vi "SubVI ATI.vi"() -> ()   [LabVIEW 2021]
uses:
  ctlSeqFNs_SubVI ATI.ctl
  ctlPkgATI.ctl
  ctlTrialState.ctl
  ctlSeqFNs.ctl
  ctlSeqFNs_SubVI PhaseSpace.ctl
  <vilib>/Analysis/Matrix/Datatypes/RealMatrix.ctl
  ctlRecording.ctl
  <vilib>/DAQmx/read.llb/DAQmx Read (Analog 2D DBL NChan NSamp).vi
  <vilib>/Analysis/baseanly.llb/Real A x B.vi
  <vilib>/Analysis/baseanly.llb/Mean (DBL).vi
  GLOBAL -MAIN.vi
  <vilib>/DAQmx/configure/trigger.llb/DAQmx Start Trigger (Digital Edge).vi
  <vilib>/DAQmx/miscellaneous.llb/DAQmx Fill In Error Info.vi
  <vilib>/Analysis/Matrix/Numeric/Conversions/Array To Matrix - RA2.vi
  <vilib>/Analysis/Matrix/Numeric/Conversions/Matrix To Array - RM.vi
  <vilib>/Analysis/Matrix/NI_Matrix.lvlib
  <resource>/objmgr/daqmx.rc
  <vilib>/Analysis/NI_AALBase.lvlib
panel:
  out "ATI plot 4":dbl[][](graph)
  out "ATI plot 3":dbl[][](graph)
  out "ATI plot 2":dbl[][](graph)
  out "ATI plot 1":dbl[][](graph)
  in  "Calib Files - TShape":path[](array[path])=[path "C:/ATI Calib files/FT8610.cal", path "C:/ATI Calib files/FT9244.cal"]
  in  "UShape?":bool
  out "Hz":dbl(graph)
  in  "Calib files - UShape":T1={"Calibration Files 1"=[path "Z:/Yen/ATI Calib files/FT8610.cal"], "Calibration Files 2"=[path "Z:/Yen/ATI Calib files/FT9244.cal"], "Calibration Files 3"=[path "Z:/Yen/ATI Calib files/FT5076.cal"], "Calibration Files 4"=[path "Z:/Yen/ATI Calib files/FT11787.cal"]}
  out "Bias":dbl[][](array[numeric]) format="%#.2f"
  in  "Bias":bool
  in  "Calib":bool
  out "save file":path
  in  "Read Cycle Time (s)":dbl=0.1 min=0.01 max=10.0 step=0.01 format="%.2f"
  out "recording?":bool
  in  "STOP":bool
  # "Parallel SubVI ATI"
  # "Acquires ATI data and Trigger signal\nSaves TDMS file."
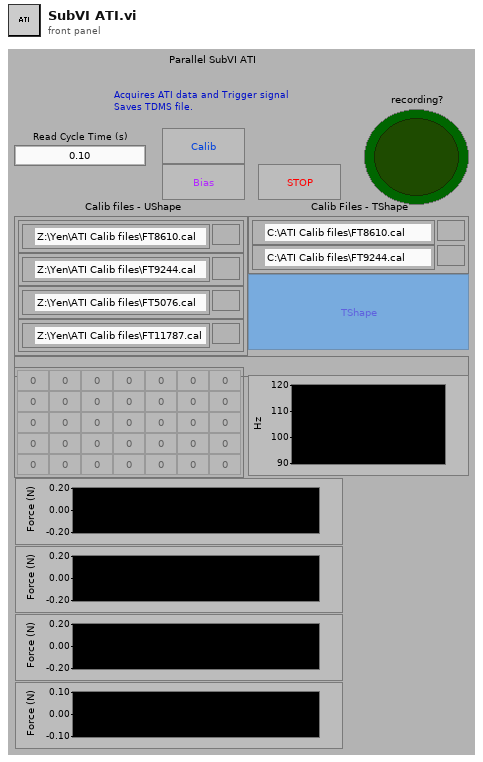
[diagram p1: front panel]
types:
  T1 = cluster{"Calibration Files 1":path[], "Calibration Files 2":path[], "Calibration Files 3":path[], "Calibration Files 4":path[]}
  T2 = typedef "ctlPkgATI.ctl" = cluster{"VIRef":refnum<vi>, "ATI":refnum<k34>, "tick ini":i64, "Trigger events":T3, "connected to server?":bool, "MAIN":refnum<queue>, "PhaseSpace":refnum<queue>, "recording?":bool, "Bias":dbl[][], "DAQmx":refnum<k21>[], "CalibMatrix":cluster{"Real Matrix":T4}[], "Data":cluster{dbl[][]}[], "tick pre":i64, "ATI Ch Names 1":string[], "ATI Ch Names 2":string[], "ATI Ch Names 3":string[], "ATI Ch Names 4":string[], "UShape?":bool}
  T3 = typedef "ctlTrialState.ctl" = enum16{"no events", "ready", "start", "hold", "stop", "end"}
  T4 = typedef "NI_Matrix.lvlib/RealMatrix.ctl" = dbl[][]
  T5 = typedef "ctlSeqFNs_SubVI ATI.ctl" = enum16{"INITIALIZE", "SET HANDLE", "IDLE", "READY", "SEND2MAIN", "CALIB Load", "BIAS", "TRIGGER", "END", "ERROR", "EXIT"}
  T6 = typedef "ctlSeqFNs.ctl" = enum16{"INITIALIZE MAIN", "UpdateProtocol", "UpdateBlockInfo", "UpdatePath", "INITIALIZE Sub", "IDLE", "Bias", "Ready", "RepeatTrial", "Events", "Get PS bias", "Get PhaseSpace", "Get ATI", "Finish", "End PhaseSpace", "End ATI", "ERROR", "EXIT"}
  T7 = typedef "ctlSeqFNs_SubVI PhaseSpace.ctl" = enum16{"INITIALIZE", "IDLE", "BIAS", "READY", "SEND2MAIN", "LOG2TDMS", "TRIGGER", "END", "ERROR", "EXIT"}
  T8 = enum16{"ALIGN -CENTER", "ALIGN -TOP LEFT", "ALIGN -AS IS", "ALIGN -CUSTOM"}
  T9 = typedef "ctlRecording.ctl" = cluster{"recording?":bool, "tdms file":refnum<k34>}
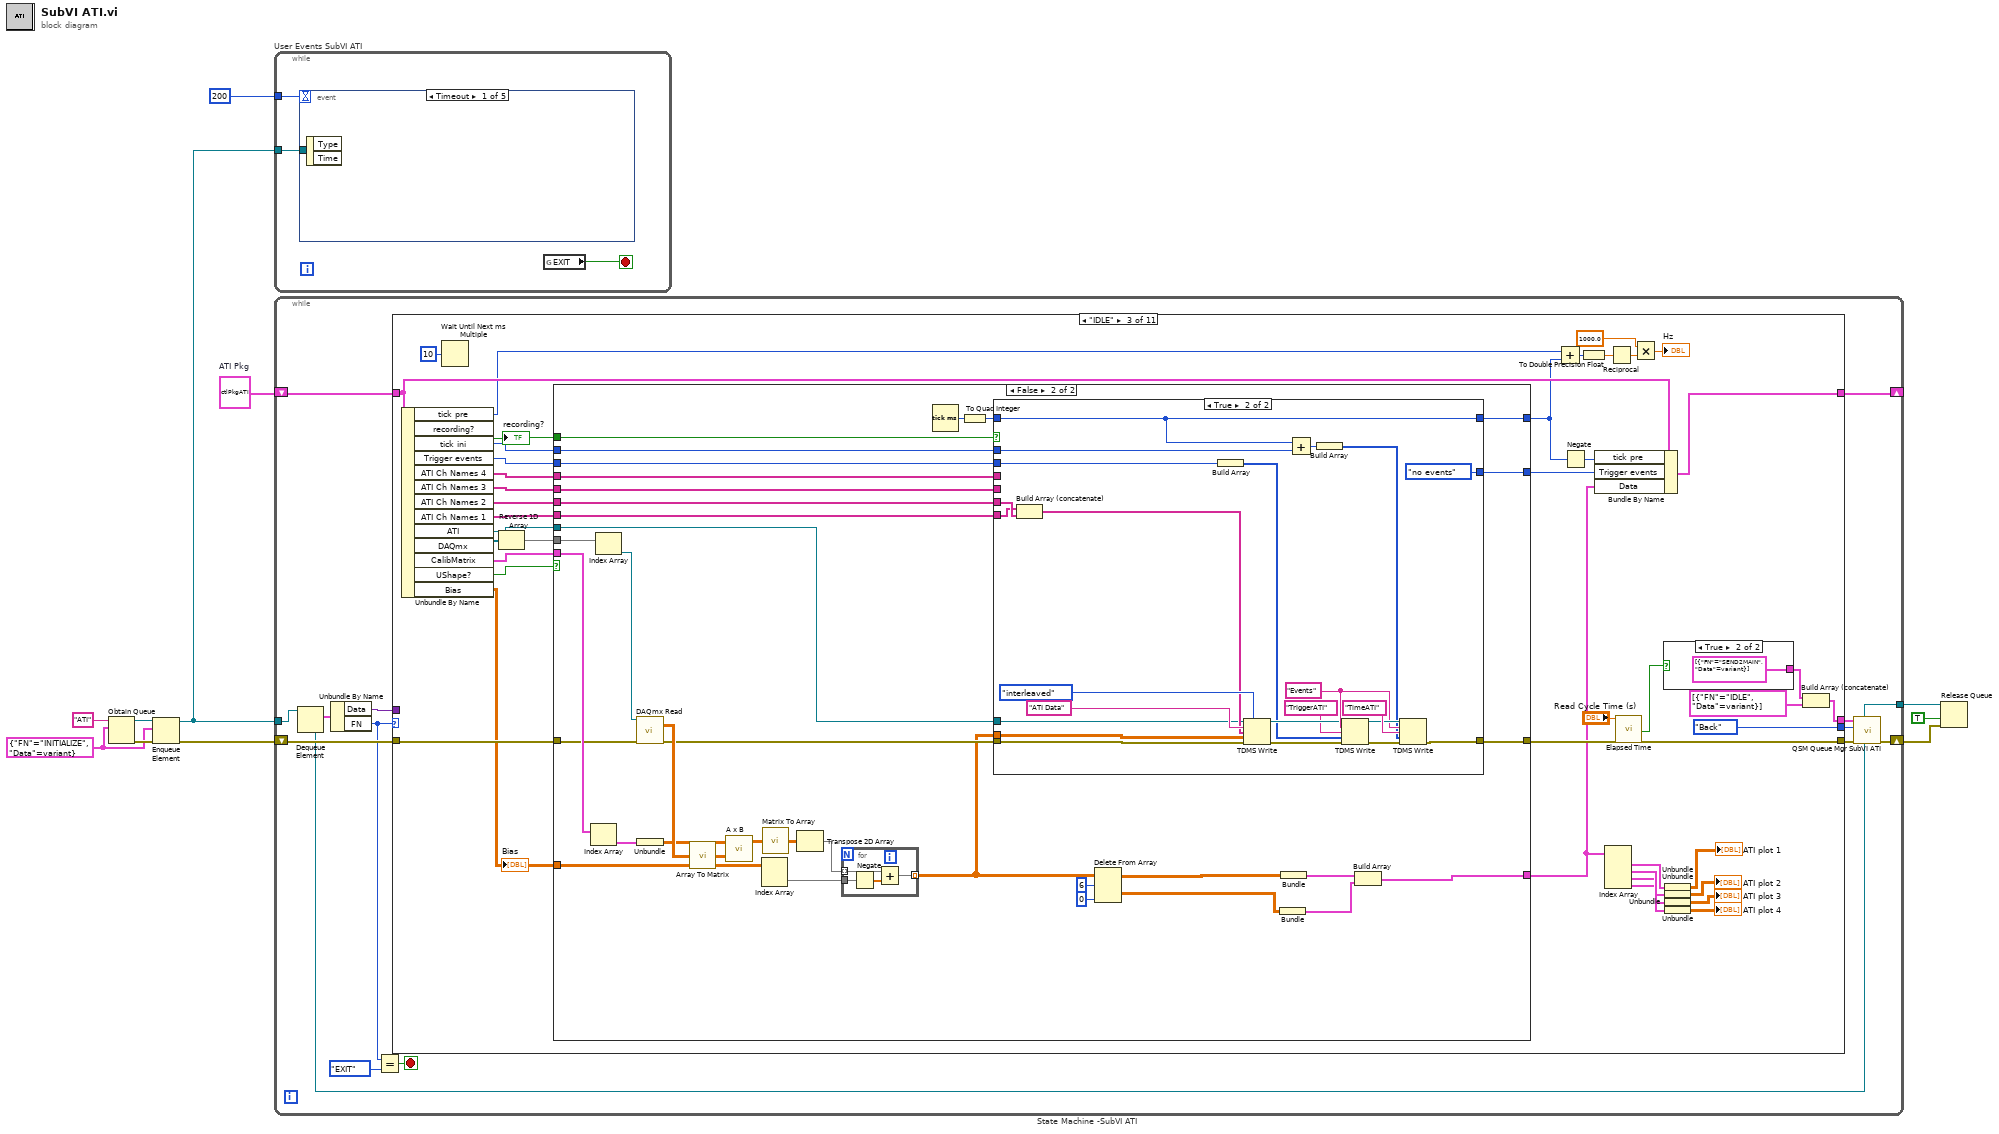
[diagram p0: block diagram]
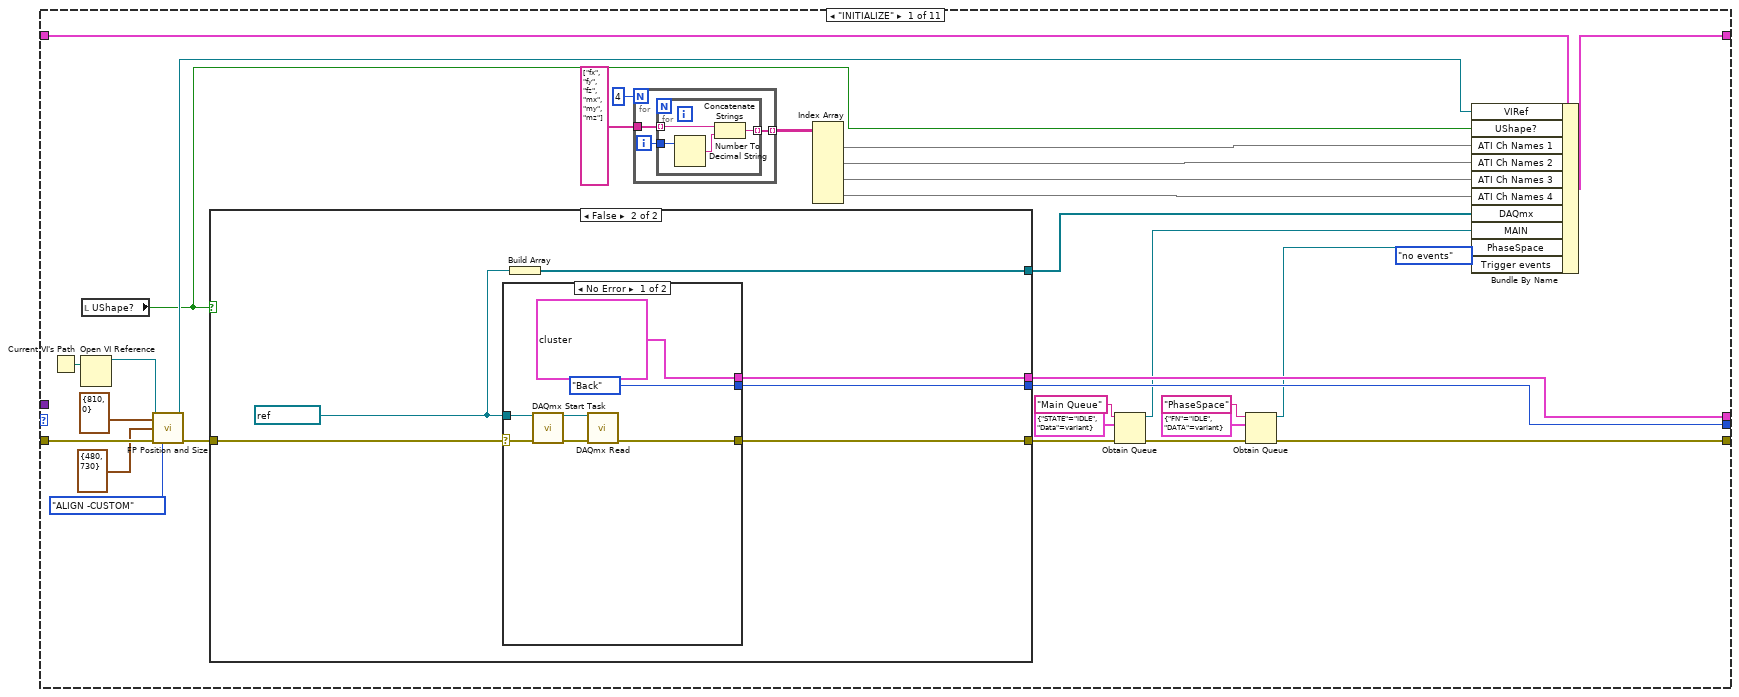
[diagram p2: hidden frame]
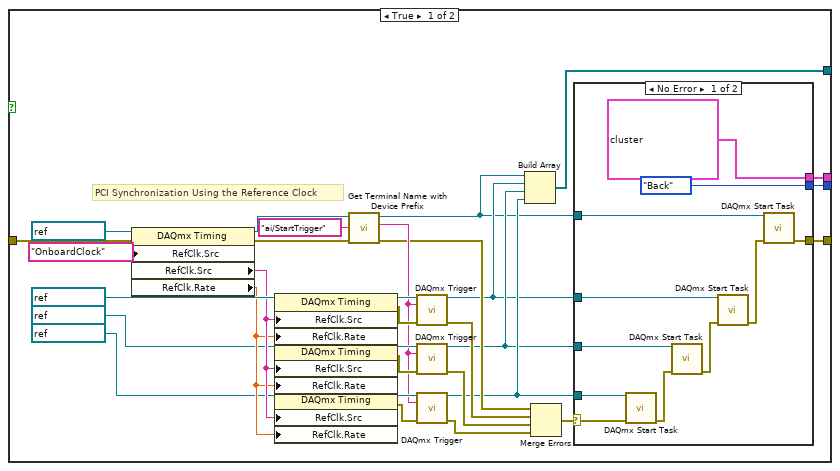
[diagram p3: hidden frame]
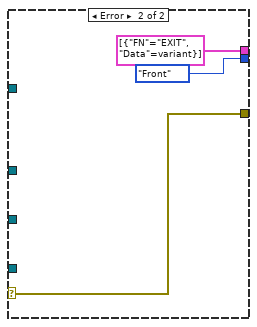
[diagram p4: hidden frame]
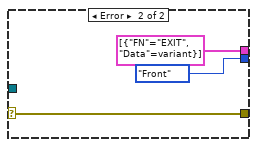
[diagram p5: hidden frame]
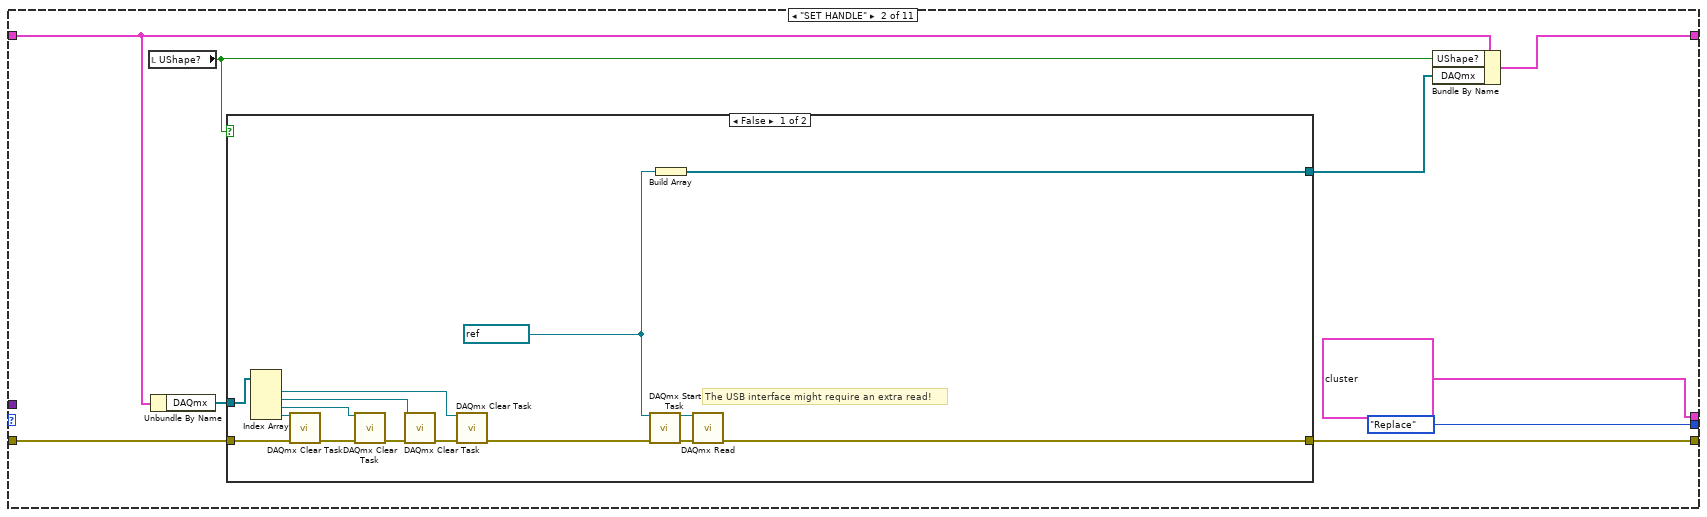
[diagram p6: hidden frame]
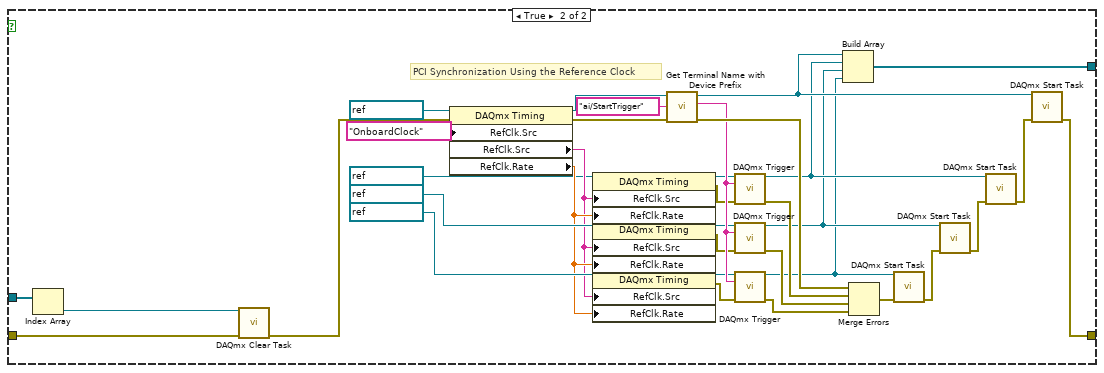
[diagram p7: hidden frame]
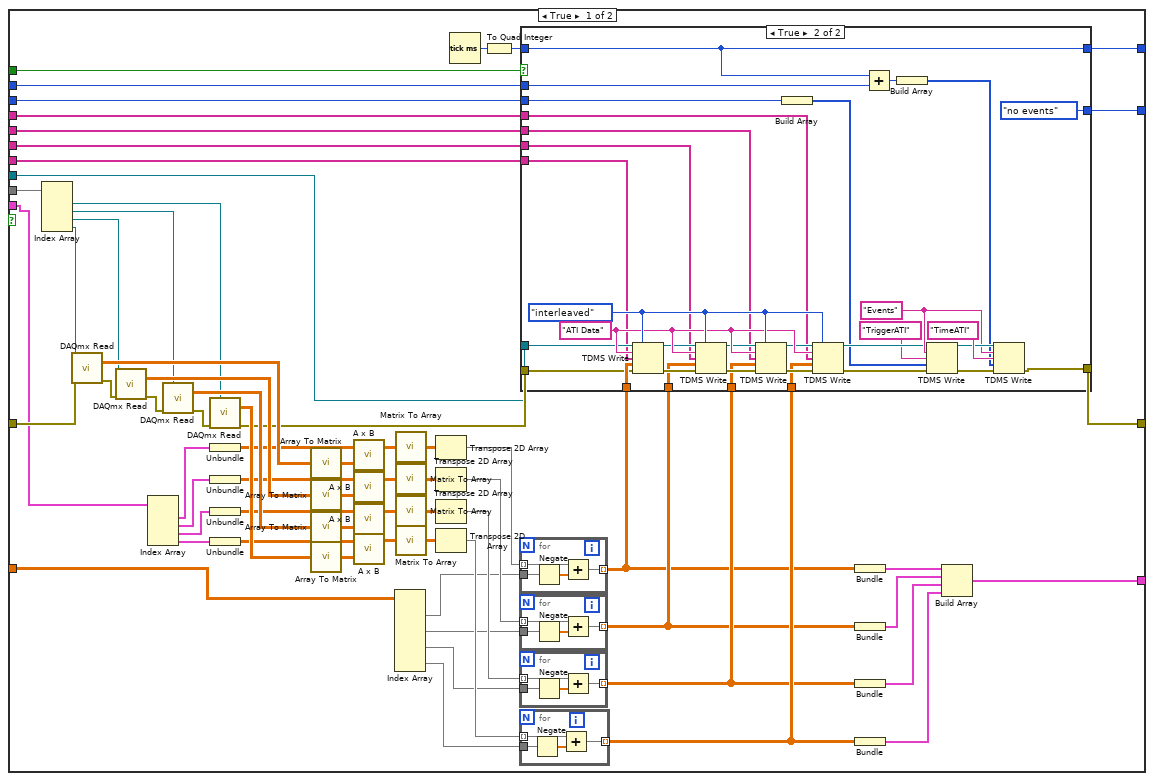
[diagram p8: hidden frame]
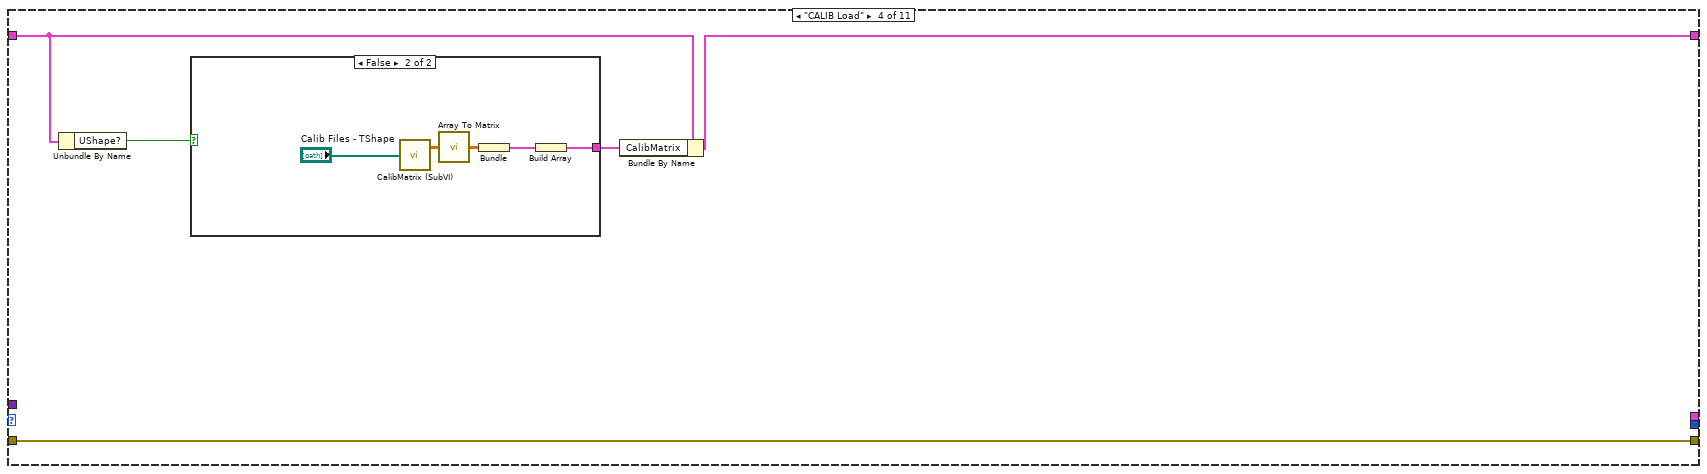
[diagram p12: hidden frame]
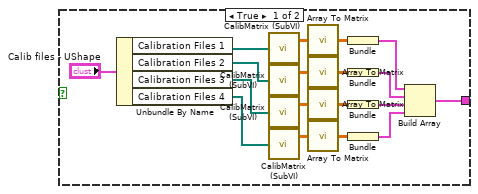
[diagram p13: hidden frame]
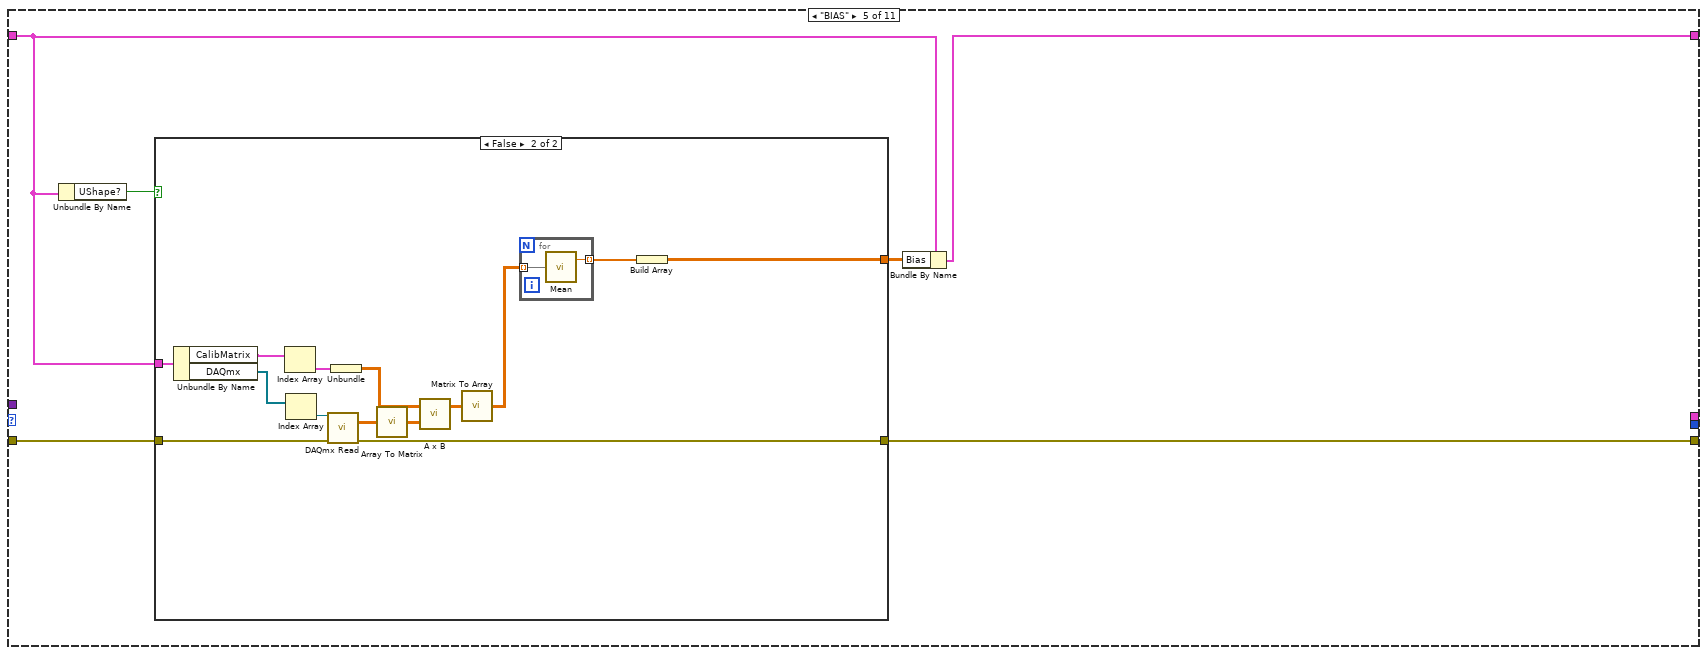
[diagram p14: hidden frame]
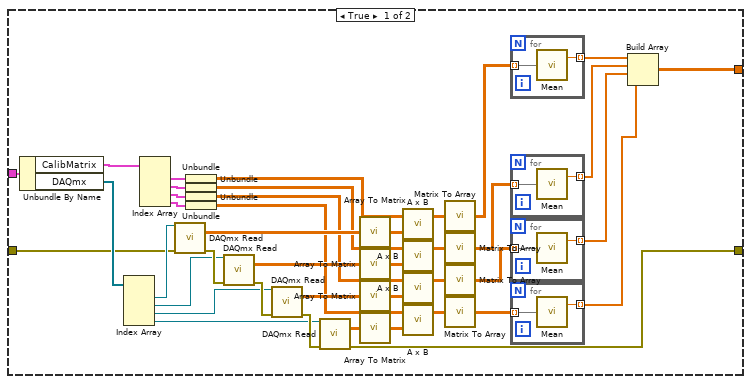
[diagram p15: hidden frame]
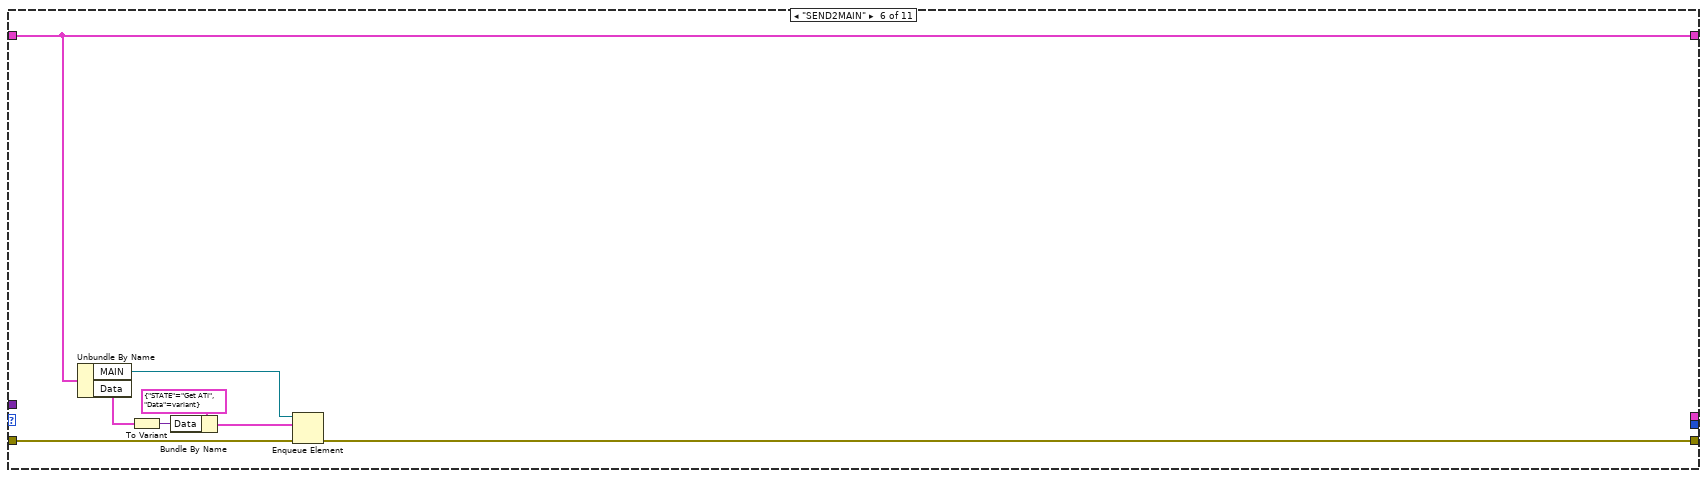
[diagram p16: hidden frame]
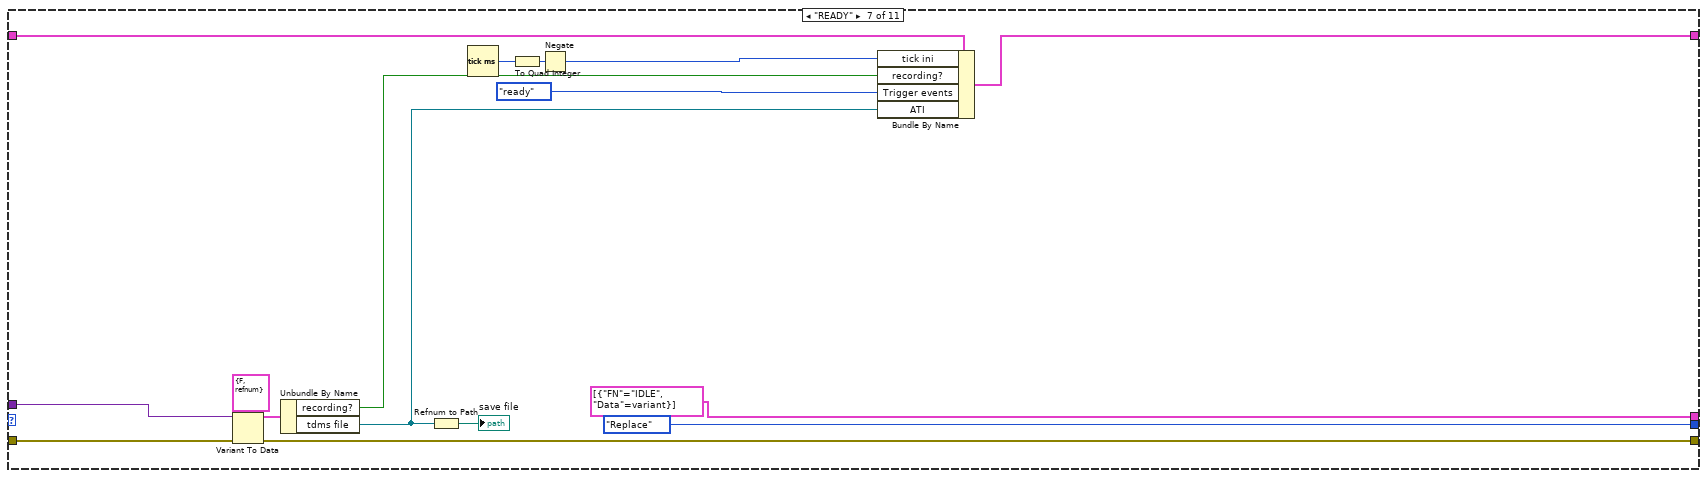
[diagram p17: hidden frame]
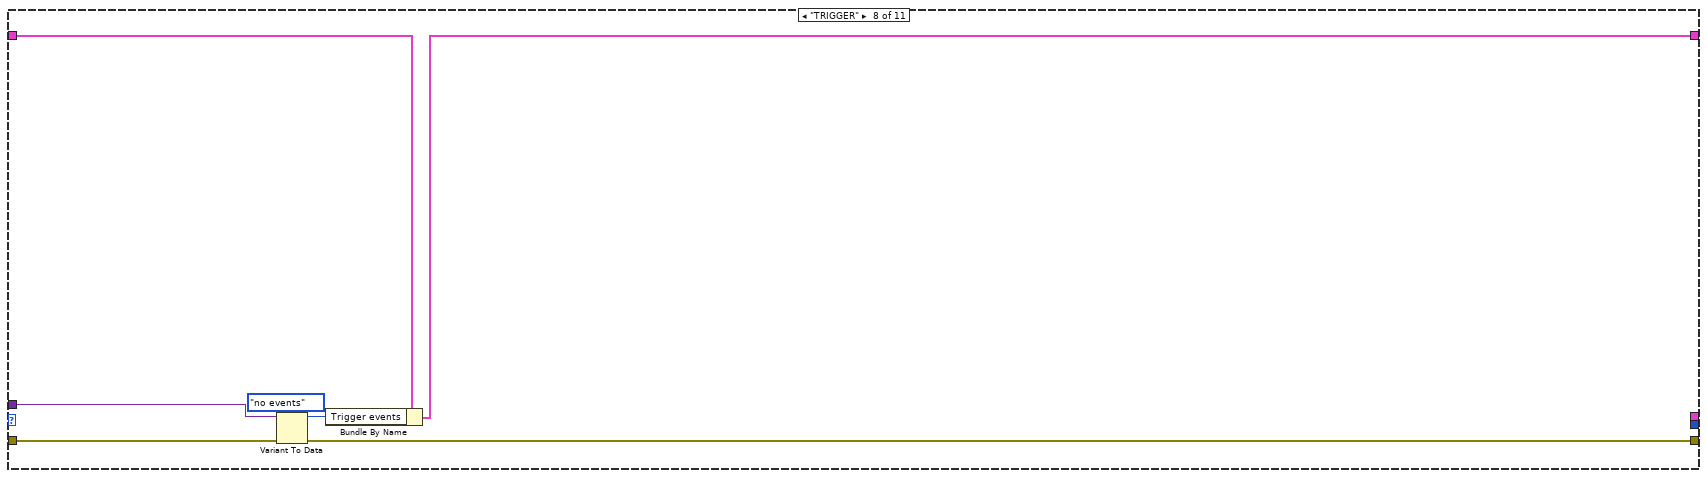
[diagram p18: hidden frame]
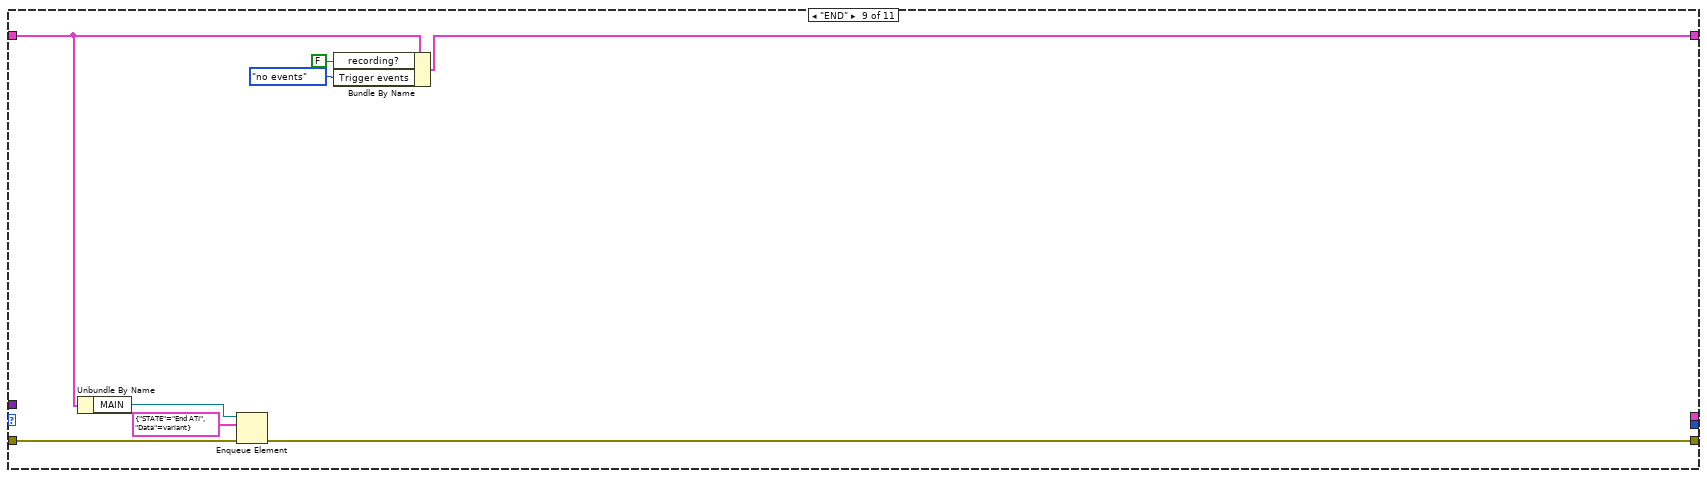
[diagram p19: hidden frame]
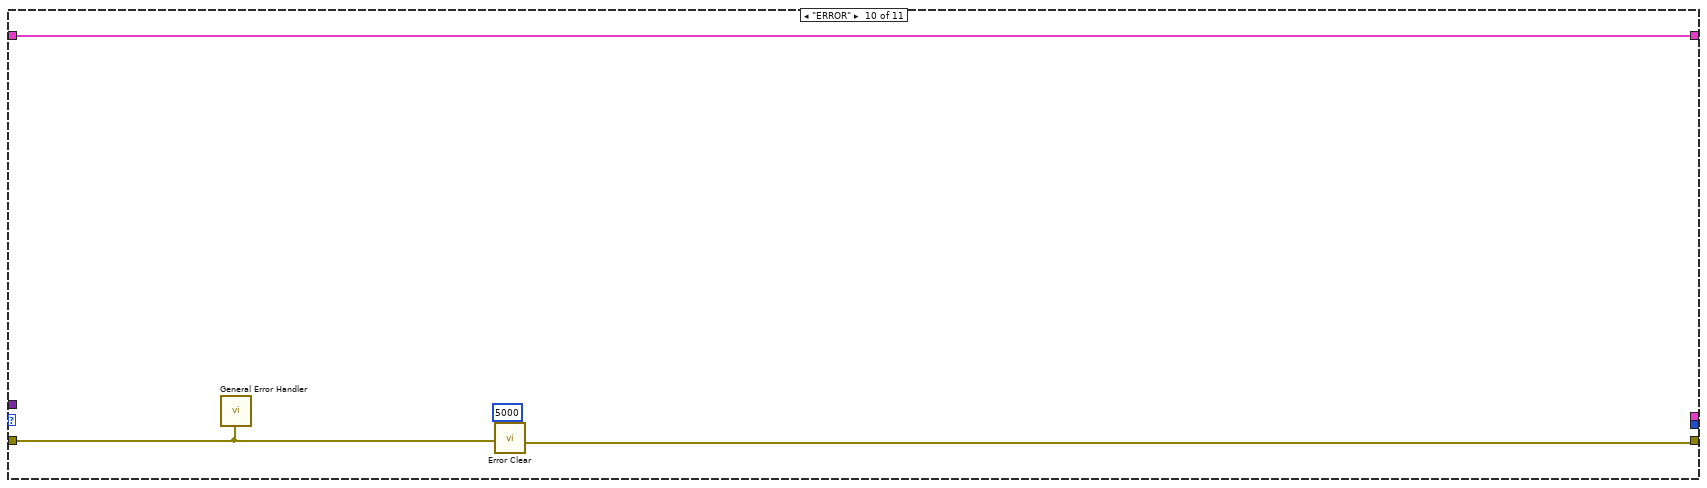
[diagram p20: hidden frame]
diagram:
  w2 = T2 {"VIRef"=refnum, "ATI"=refnum, "tick ini"=0, "Trigger events"=enum."no events", "connected to server?"=FALSE, "MAIN"=refnum, "PhaseSpace"=refnum, "recording?"=FALSE, "Bias"=[], "DAQmx"=[], "CalibMatrix"=[], "Data"=[], "tick pre"=0, "ATI Ch Names 1"=[], "ATI Ch Names 2"=[], "ATI Ch Names 3"=[], "ATI Ch Names 4"=[], "UShape?"=FALSE}  # ATI Pkg
  w6 = cluster{"FN":T5, "Data":variant} {"FN"=enum."INITIALIZE", "Data"=variant} ("cluFNData")
  n1 = Obtain Queue(name (unnamed)="ATI", element data type=w6) -> (queue out=w7:refnum<queue>, error out=w9:errorcluster)  [unwired: 3 in, 1 out]
  n2 = Enqueue Element(queue=w7, element=w6, error in (no error)=w9) -> (queue out=w3:refnum<queue>, error out=w8:errorcluster)  [unwired: 1 in, 1 out]
  n3 = while "User Events SubVI ATI" {
    tunnel: 200 -> [w14]
    tunnel: w3 -> [w12]
    stop <- w13 stop-if-true
    n4 = event shown="[0] Timeout" {
      selector: _ -> [_ _ _ _ _]
      dyn-events: _ -> [_ _ _ _ _]
      timeout: w14 -> [_ _ _ _ _]
      tunnel: w12 -> [_ w16 w18 w20 w22]
      event Timeout {
        n5 = event-data() -> ()  [unwired: 1 in, 2 out]
      }
      event "STOP": Value Change {
        n6 = event-data() -> ()  [unwired: 1 in, 1 out]
        n7 = Enqueue Element(queue=w16, element=cluster{"FN":T5, "Data":variant} {"FN"=enum."EXIT", "Data"=variant}) -> ()  [unwired: 2 in, 3 out]
      }
      event "Calib": Value Change {
        n8 = event-data() -> ()  [unwired: 1 in, 1 out]
        n9 = Enqueue Element(queue=w18, element=cluster{"FN":T5, "Data":variant} {"FN"=enum."CALIB Load", "Data"=variant}) -> ()  [unwired: 2 in, 3 out]
      }
      event "Bias": Value Change {
        n10 = event-data() -> ()  [unwired: 1 in, 1 out]
        n11 = Enqueue Element(queue=w20, element=cluster{"FN":T5, "Data":variant} {"FN"=enum."BIAS", "Data"=variant}) -> ()  [unwired: 2 in, 3 out]
      }
      event "UShape?": Value Change {
        n12 = event-data() -> ()  [unwired: 1 in, 2 out]
        n13 = Enqueue Element(queue=w22, element=cluster{"FN":T5, "Data":variant} {"FN"=enum."SET HANDLE", "Data"=variant}) -> ()  [unwired: 2 in, 3 out]
      }
    }
    n14 = global read "GLOBAL -MAIN.vi" "EXIT"() -> (w13:bool)
  }
  n15 = while "State Machine -SubVI ATI" {
    shift-right: [w26] -> w1
    shift-left: w8 -> [w36]
    tunnel: w3 -> [w33]
    tunnel: [w24] -> w5
    shift-right: [w28] -> _
    shift-left: w2 -> [w29]
    stop <- w35 stop-if-true
    n16 = Dequeue Element(queue=w33) -> (queue out=w24:refnum<queue>, element=w32:cluster{"FN":T5, "Data":variant})  [unwired: 2 in, 2 out]
    n17 = Unbundle By Name(w32) -> ("Data"=w31:variant, "FN"=w30:T5)
    n18 = Equal?(x=w30, y=ctlSeqFNs_SubVI_ATI."EXIT" ("FN")) -> (x = y?=w35:bool)
    n19 = case shown="\"IDLE\"" w30 {
      tunnel: w36 -> [w65 w142 w227 w425 w453 w528 w533 w551 w553 w560 w567]
      tunnel: [w61 w141 w229 w425 w452 w527 w539 w550 w552 w562 w569] -> w27
      tunnel: w31 -> [_ _ _ _ _ _ w540 w549 _ _ _]
      tunnel: w29 -> [w57 w140 w226 w423 w451 w526 w535 w547 w555 w563 w566]
      tunnel: [w48 w144 w228 w426 w455 w526 w544 w548 w559 w563 w566] -> w28
      tunnel: [w56 cluster{"FN":T5, "Data":variant}[] [{"FN"=enum."CALIB Load", "Data"=variant}, {"FN"=enum."BIAS", "Data"=variant}, {"FN"=enum."IDLE", "Data"=variant}] ("QFNs") w233 _ _ _ cluster{"FN":T5, "Data":variant}[] [{"FN"=enum."IDLE", "Data"=variant}] ("QFNs") _ _ _ _] -> w23
      tunnel: [w55 enum16{"Back", "Front", "Replace"}."Replace" ("Enum") enum16{"Back", "Front", "Replace"}."Back" ("Enum") _ _ _ enum16{"Back", "Front", "Replace"}."Replace" ("Enum") _ _ _ _] -> w25
      frame "INITIALIZE" {
        n20 = Current VI's Path() -> (path=w67:path)
        n21 = Open VI Reference(vi path=w67) -> (vi reference=w66:refnum<vi>)  [unwired: 5 in, 1 out]
        n22 = local read "UShape?"() -> (w37:bool)
        n23 = call "FP Position and Size.vi"("VIRefNum  IN"=w66, "Poistion"=cluster{"left":i16, "top":i16} {"left"=810, "top"=0}, "Size"=cluster{"right":i16, "bottom":i16} {"right"=480, "bottom"=730}, "error in (no error)"=w65, "Mode"=T8."ALIGN -CUSTOM") -> ("VIRefNum OUT"=w38:refnum<vi>, "error out"=w51:errorcluster)  [unwired: 9 in]
        n24 = case shown="False" w37 {
          tunnel: [w98 w118] -> w58
          tunnel: [w97 w117] -> w56
          tunnel: [w96 w116] -> w55
          tunnel: w51 -> [w74 w114]
          tunnel: [w68 w115] -> w39
          frame True {
            # "PCI Synchronization Using the Reference Clock"
            n25 = property class="DAQmx Timing"(reference=refnum<k21> "UShape1" ("DAQmx Task Name"), error in=w74, "RefClk.Src"=tag "OnboardClock") -> (reference out=w88:refnum<k21>, error out=w86:errorcluster, "RefClk.Src"=w92:tag, "RefClk.Rate"=w91:dbl)
            n26 = property class="DAQmx Timing"(reference=refnum<k21> "UShape2" ("DAQmx Task Name"), "RefClk.Src"=w92, "RefClk.Rate"=w91) -> (reference out=w85:refnum<k21>, error out=w84:errorcluster)  [unwired: 1 in]
            n27 = property class="DAQmx Timing"(reference=refnum<k21> "UShape3" ("DAQmx Task Name"), "RefClk.Src"=w92, "RefClk.Rate"=w91) -> (reference out=w83:refnum<k21>, error out=w82:errorcluster)  [unwired: 1 in]
            n28 = property class="DAQmx Timing"(reference=refnum<k21> "UShape4" ("DAQmx Task Name"), "RefClk.Src"=w92, "RefClk.Rate"=w91) -> (reference out=w81:refnum<k21>, error out=w80:errorcluster)  [unwired: 1 in]
            n29 = call "Get Terminal Name with Device Prefix.vi"("error in (no error)"=w86, "Local Terminal Name"="ai/StartTrigger", "task/channels in"=w88) -> ("error out"=w78:errorcluster, "Terminal Name with Device Prefix"=w79:tag, "task out"=w69:refnum<k21>)  [unwired: 6 in]
            n30 = call-poly <vilib>:"DAQmx Trigger.vi"("task/channels in"=w85, "source"=w79, "error in"=w84) -> ("task out"=w70:refnum<k21>, "error out"=w77:errorcluster)  [unwired: 11 in]
            n31 = call-poly <vilib>:"DAQmx Trigger.vi"("task/channels in"=w83, "source"=w79, "error in"=w82) -> ("task out"=w71:refnum<k21>, "error out"=w76:errorcluster)  [unwired: 11 in]
            n32 = call-poly <vilib>:"DAQmx Trigger.vi"("task/channels in"=w81, "source"=w79, "error in"=w80) -> ("task out"=w72:refnum<k21>, "error out"=w75:errorcluster)  [unwired: 11 in]
            n33 = Build Array(w69, w70, w71, w72) -> (w68:refnum<k21>[])
            n34 = Merge Errors(w78, w77, w76, w75) -> (w73:errorcluster)
            n35 = case shown="No Error" w73 {
              selector: w73 -> [w104 w112]
              tunnel: [w103 w112] -> w98
              tunnel: [cluster{"FN":T5, "Data":variant}[] [{"FN"=enum."CALIB Load", "Data"=variant}, {"FN"=enum."BIAS", "Data"=variant}, {"FN"=enum."IDLE", "Data"=variant}] ("QFNs") cluster{"FN":T5, "Data":variant}[] [{"FN"=enum."EXIT", "Data"=variant}] ("QFNs")] -> w97
              tunnel: [enum16{"Back", "Front", "Replace"}."Back" ("Enum") enum16{"Back", "Front", "Replace"}."Front" ("Enum")] -> w96
              tunnel: w72 -> [w102 _]
              tunnel: w71 -> [w101 _]
              tunnel: w70 -> [w100 _]
              tunnel: w69 -> [w99 _]
              frame No Error {
                n36 = call <vilib>:"DAQmx Start Task.vi"("task/channels in"=w102, "error in"=w104) -> ("error out"=w107:errorcluster)  [unwired: 12 in, 1 out]
                n37 = call <vilib>:"DAQmx Start Task.vi"("task/channels in"=w101, "error in"=w107) -> ("error out"=w106:errorcluster)  [unwired: 12 in, 1 out]
                n38 = call <vilib>:"DAQmx Start Task.vi"("task/channels in"=w100, "error in"=w106) -> ("error out"=w105:errorcluster)  [unwired: 12 in, 1 out]
                n39 = call <vilib>:"DAQmx Start Task.vi"("task/channels in"=w99, "error in"=w105) -> ("error out"=w103:errorcluster)  [unwired: 12 in, 1 out]
              }
              frame Error {
              }
            }
          }
          frame False {
            w113 = refnum<k21> "TShape" ("DAQmx Task Name")
            n40 = case shown="No Error" w114 {
              selector: w114 -> [w121 w128]
              tunnel: [w120 w128] -> w118
              tunnel: [cluster{"FN":T5, "Data":variant}[] [{"FN"=enum."CALIB Load", "Data"=variant}, {"FN"=enum."BIAS", "Data"=variant}, {"FN"=enum."IDLE", "Data"=variant}] ("QFNs") cluster{"FN":T5, "Data":variant}[] [{"FN"=enum."EXIT", "Data"=variant}] ("QFNs")] -> w117
              tunnel: [enum16{"Back", "Front", "Replace"}."Back" ("Enum") enum16{"Back", "Front", "Replace"}."Front" ("Enum")] -> w116
              tunnel: w113 -> [w122 _]
              frame No Error {
                n41 = call <vilib>:"DAQmx Start Task.vi"("task/channels in"=w122, "error in"=w121) -> ("task out"=w119:refnum<k21>, "error out"=w123:errorcluster)  [unwired: 12 in]
                n42 = call-poly <vilib>:"DAQmx Read.vi"("task/channels in"=w119, "error in"=w123) -> ("error out"=w120:errorcluster)  [unwired: 11 in, 2 out]
              }
              frame Error {
              }
            }
            n43 = Build Array(w113) -> (w115:refnum<k21>[])
          }
        }
        n44 = for {
          N: 4 -> [_]
          tunnel: string[] ["fx", "fy", "fz", "mx", "my", "mz"] -> [w131]
          tunnel: [w129] -> w44 mode=indexing
          i -> [w130]
          n45 = for {
            tunnel: w131 -> [w135] mode=indexing
            tunnel: w130 -> [w134]
            tunnel: [w132] -> w129 mode=indexing
            n46 = Number To Decimal String(number=w134) -> (decimal integer string=w133:string)  [unwired: 1 in]
            n47 = Concatenate Strings(w135, w133) -> (w132:string)
          }
        }
        n48 = Index Array(array=w44) -> (element #1=w40:string[], element #2=w41:string[], element #3=w42:string[], element #4=w43:string[])  [unwired: 8 in]
        n49 = Obtain Queue(name (unnamed)="Main Queue", element data type=cluster{"STATE":T6, "Data":variant} {"STATE"=enum."IDLE", "Data"=variant} ("element"), error in (no error)=w58) -> (queue out=w50:refnum<queue>, error out=w54:errorcluster)  [unwired: 2 in, 1 out]
        n50 = Obtain Queue(name (unnamed)="PhaseSpace", element data type=cluster{"FN":T7, "DATA":variant} {"FN"=enum."IDLE", "DATA"=variant} ("cluFNData"), error in (no error)=w54) -> (queue out=w49:refnum<queue>, error out=w61:errorcluster)  [unwired: 2 in, 1 out]
        n51 = Bundle By Name(cluster=w57, "VIRef"=w38, "UShape?"=w37, "ATI Ch Names 1"=w40, "ATI Ch Names 2"=w41, "ATI Ch Names 3"=w42, "ATI Ch Names 4"=w43, "DAQmx"=w39, "MAIN"=w50, "PhaseSpace"=w49, "Trigger events"=ctlTrialState."no events") -> (w48:T2)
      }
      frame "SET HANDLE" {
        n52 = local read "UShape?"() -> (w137:bool)
        n53 = Unbundle By Name(w140) -> ("DAQmx"=w143:refnum<k21>[])
        n54 = case shown="False" w137 {
          tunnel: [w146 w163] -> w141
          tunnel: w142 -> [w148 w160]
          tunnel: w143 -> [w156 w194]
          tunnel: [w153 w172] -> w139
          frame False {
            w155 = refnum<k21> "TShape" ("DAQmx Task Name")
            # "The USB interface might require an extra read!"
            n55 = Index Array(array=w156) -> (element #1=w152:refnum<k21>, element #2=w151:refnum<k21>, element #3=w150:refnum<k21>, element #4=w149:refnum<k21>)  [unwired: 4 in]
            n56 = call <vilib>:"DAQmx Clear Task.vi"("task in"=w149, "error in"=w148) -> ("error out"=w159:errorcluster)  [unwired: 13 in]
            n57 = call <vilib>:"DAQmx Clear Task.vi"("task in"=w150, "error in"=w159) -> ("error out"=w158:errorcluster)  [unwired: 13 in]
            n58 = call <vilib>:"DAQmx Clear Task.vi"("task in"=w151, "error in"=w158) -> ("error out"=w157:errorcluster)  [unwired: 13 in]
            n59 = call <vilib>:"DAQmx Clear Task.vi"("task in"=w152, "error in"=w157) -> ("error out"=w154:errorcluster)  [unwired: 13 in]
            n60 = call <vilib>:"DAQmx Start Task.vi"("task/channels in"=w155, "error in"=w154) -> ("task out"=w145:refnum<k21>, "error out"=w147:errorcluster)  [unwired: 12 in]
            n61 = Build Array(w155) -> (w153:refnum<k21>[])
            n62 = call-poly <vilib>:"DAQmx Read.vi"("task/channels in"=w145, "error in"=w147) -> ("error out"=w146:errorcluster)  [unwired: 11 in, 2 out]
          }
          frame True {
            # "PCI Synchronization Using the Reference Clock"
            n63 = Index Array(array=w194) -> (element=w161:refnum<k21>)  [unwired: 1 in]
            n64 = call <vilib>:"DAQmx Clear Task.vi"("task in"=w161, "error in"=w160) -> ("error out"=w162:errorcluster)  [unwired: 13 in]
            n65 = property class="DAQmx Timing"(reference=refnum<k21> "UShape1" ("DAQmx Task Name"), error in=w162, "RefClk.Src"=tag "OnboardClock") -> (reference out=w180:refnum<k21>, error out=w182:errorcluster, "RefClk.Src"=w176:tag, "RefClk.Rate"=w177:dbl)
            n66 = property class="DAQmx Timing"(reference=refnum<k21> "UShape2" ("DAQmx Task Name"), "RefClk.Src"=w176, "RefClk.Rate"=w177) -> (reference out=w183:refnum<k21>, error out=w184:errorcluster)  [unwired: 1 in]
            n67 = property class="DAQmx Timing"(reference=refnum<k21> "UShape3" ("DAQmx Task Name"), "RefClk.Src"=w176, "RefClk.Rate"=w177) -> (reference out=w185:refnum<k21>, error out=w186:errorcluster)  [unwired: 1 in]
            n68 = property class="DAQmx Timing"(reference=refnum<k21> "UShape4" ("DAQmx Task Name"), "RefClk.Src"=w176, "RefClk.Rate"=w177) -> (reference out=w187:refnum<k21>, error out=w188:errorcluster)  [unwired: 1 in]
            n69 = call "Get Terminal Name with Device Prefix.vi"("error in (no error)"=w182, "Local Terminal Name"="ai/StartTrigger", "task/channels in"=w180) -> ("error out"=w190:errorcluster, "Terminal Name with Device Prefix"=w189:tag, "task out"=w168:refnum<k21>)  [unwired: 6 in]
            n70 = call-poly <vilib>:"DAQmx Trigger.vi"("task/channels in"=w183, "source"=w189, "error in"=w184) -> ("task out"=w167:refnum<k21>, "error out"=w191:errorcluster)  [unwired: 11 in]
            n71 = call-poly <vilib>:"DAQmx Trigger.vi"("task/channels in"=w185, "source"=w189, "error in"=w186) -> ("task out"=w166:refnum<k21>, "error out"=w192:errorcluster)  [unwired: 11 in]
            n72 = call-poly <vilib>:"DAQmx Trigger.vi"("task/channels in"=w187, "source"=w189, "error in"=w188) -> ("task out"=w165:refnum<k21>, "error out"=w193:errorcluster)  [unwired: 11 in]
            n73 = Build Array(w168, w167, w166, w165) -> (w172:refnum<k21>[])
            n74 = Merge Errors(w190, w191, w192, w193) -> (w164:errorcluster)
            n75 = call <vilib>:"DAQmx Start Task.vi"("task/channels in"=w165, "error in"=w164) -> ("error out"=w169:errorcluster)  [unwired: 12 in, 1 out]
            n76 = call <vilib>:"DAQmx Start Task.vi"("task/channels in"=w166, "error in"=w169) -> ("error out"=w170:errorcluster)  [unwired: 12 in, 1 out]
            n77 = call <vilib>:"DAQmx Start Task.vi"("task/channels in"=w167, "error in"=w170) -> ("error out"=w171:errorcluster)  [unwired: 12 in, 1 out]
            n78 = call <vilib>:"DAQmx Start Task.vi"("task/channels in"=w168, "error in"=w171) -> ("error out"=w163:errorcluster)  [unwired: 12 in, 1 out]
          }
        }
        n79 = Bundle By Name(cluster=w140, "UShape?"=w137, "DAQmx"=w139) -> (w144:T2)
      }
      frame "IDLE" {
        n80 = Unbundle By Name(w226) -> ("tick pre"=w211:i64, "recording?"=w204:bool, "tick ini"=w212:i64, "Trigger events"=w213:T3, "ATI Ch Names 4"=w208:string[], "ATI Ch Names 3"=w209:string[], "ATI Ch Names 2"=w210:string[], "ATI Ch Names 1"=w224:string[], "ATI"=w220:refnum<k34>, "DAQmx"=w221:refnum<k21>[], "CalibMatrix"=w222:cluster{"Real Matrix":T4}[], "UShape?"=w206:bool, "Bias"=w205:dbl[][])
        "Bias" <- w205
        "recording?" <- w204
        n81 = Wait Until Next ms Multiple(millisecond multiple=u32 10) -> ()  [unwired: 1 out]
        n82 = Reverse 1D Array(array=w221) -> (reversed array=w225:refnum<k21>[])
        n83 = case shown="False" w206 {
          tunnel: [w303 w390] -> w230
          tunnel: w227 -> [w279 w364]
          tunnel: w225 -> [w277 w383]
          tunnel: w224 -> [w268 w381]
          tunnel: [w255 w378] -> w195
          tunnel: [w254 w377] -> w223
          tunnel: w205 -> [w253 w376]
          tunnel: w222 -> [w242 w365]
          tunnel: w220 -> [w252 w375]
          tunnel: [w251 w374] -> w215
          tunnel: w213 -> [w250 w373]
          tunnel: w212 -> [w249 w372]
          tunnel: w204 -> [w248 w371]
          tunnel: w210 -> [w247 w370]
          tunnel: w209 -> [w246 w369]
          tunnel: w208 -> [w245 w368]
          frame True {
            n84 = Index Array(array=w277) -> (element #1=w276:refnum<k21>, element #2=w275:refnum<k21>, element #3=w274:refnum<k21>, element #4=w273:refnum<k21>)  [unwired: 4 in]
            n85 = call-poly <vilib>:"DAQmx Read.vi"("task/channels in"=w273, "error in"=w279) -> ("data"=w297:dbl[][], "error out"=w302:errorcluster)  [unwired: 11 in, 1 out]
            n86 = call-poly <vilib>:"DAQmx Read.vi"("task/channels in"=w274, "error in"=w302) -> ("data"=w290:dbl[][], "error out"=w301:errorcluster)  [unwired: 11 in, 1 out]
            n87 = Index Array(array=w242) -> (element #1=w263:cluster{"Real Matrix":T4}, element #2=w262:cluster{"Real Matrix":T4}, element #3=w261:cluster{"Real Matrix":T4}, element #4=w260:cluster{"Real Matrix":T4})  [unwired: 4 in]
            n88 = call-poly <vilib>:"DAQmx Read.vi"("task/channels in"=w275, "error in"=w301) -> ("data"=w289:dbl[][], "error out"=w300:errorcluster)  [unwired: 11 in, 1 out]
            n89 = call-poly <vilib>:"DAQmx Read.vi"("task/channels in"=w276, "error in"=w300) -> ("data"=w288:dbl[][], "error out"=w278:errorcluster)  [unwired: 11 in, 1 out]
            n90 = Unbundle(w263) -> ("Real Matrix"=w267:T4)
            n91 = Unbundle(w262) -> ("Real Matrix"=w266:T4)
            n92 = Unbundle(w261) -> ("Real Matrix"=w265:T4)
            n93 = Unbundle(w260) -> ("Real Matrix"=w264:T4)
            n94 = call-poly <vilib>:"Array To Matrix.vi"("Real 2D Array"=w297) -> ("Real Matrix"=w299:T4)
            n95 = call-poly <vilib>:"Array To Matrix.vi"("Real 2D Array"=w290) -> ("Real Matrix"=w295:T4)
            n96 = call-poly <vilib>:"Array To Matrix.vi"("Real 2D Array"=w289) -> ("Real Matrix"=w294:T4)
            n97 = call-poly <vilib>:"Array To Matrix.vi"("Real 2D Array"=w288) -> ("Real Matrix"=w291:T4)
            n98 = call-poly <vilib>:"A x B.vi"("B"=w299, "A"=w267) -> ("A x B"=w298:T4)  [unwired: 1 out]
            n99 = call-poly <vilib>:"A x B.vi"("B"=w295, "A"=w266) -> ("A x B"=w296:T4)  [unwired: 1 out]
            n100 = call-poly <vilib>:"A x B.vi"("B"=w294, "A"=w265) -> ("A x B"=w293:T4)  [unwired: 1 out]
            n101 = call-poly <vilib>:"A x B.vi"("B"=w291, "A"=w264) -> ("A x B"=w292:T4)  [unwired: 1 out]
            n102 = Index Array(array=w253) -> (element #1=w269:dbl[], element #2=w272:dbl[], element #3=w271:dbl[], element #4=w270:dbl[])  [unwired: 8 in]
            n103 = call-poly <vilib>:"Matrix To Array.vi"("Real Matrix"=w298) -> ("Real 2D Array"=w287:dbl[][])
            n104 = call-poly <vilib>:"Matrix To Array.vi"("Real Matrix"=w296) -> ("Real 2D Array"=w286:dbl[][])
            n105 = call-poly <vilib>:"Matrix To Array.vi"("Real Matrix"=w293) -> ("Real 2D Array"=w285:dbl[][])
            n106 = call-poly <vilib>:"Matrix To Array.vi"("Real Matrix"=w292) -> ("Real 2D Array"=w284:dbl[][])
            n107 = Transpose 2D Array(2D array=w287) -> (transposed array=w283:dbl[][])
            n108 = Transpose 2D Array(2D array=w286) -> (transposed array=w282:dbl[][])
            n109 = Transpose 2D Array(2D array=w285) -> (transposed array=w281:dbl[][])
            n110 = Transpose 2D Array(2D array=w284) -> (transposed array=w280:dbl[][])
            n111 = Tick Count (ms)() -> (millisecond timer value=w244:u32)
            n112 = To Quad Integer(1:w244) -> (0:w243:i64)
            n113 = for {
              tunnel: w283 -> [w312] mode=indexing
              tunnel: w269 -> [w315]
              tunnel: [w314] -> w238 mode=indexing
              n114 = Negate(x=w315) -> (-x=w313:dbl[])
              n115 = Add(x=w312, y=w313) -> (x+y=w314:dbl[])
            }
            n116 = for {
              tunnel: w282 -> [w308] mode=indexing
              tunnel: w272 -> [w311]
              tunnel: [w310] -> w239 mode=indexing
              n117 = Negate(x=w311) -> (-x=w309:dbl[])
              n118 = Add(x=w308, y=w309) -> (x+y=w310:dbl[])
            }
            n119 = for {
              tunnel: w281 -> [w304] mode=indexing
              tunnel: w271 -> [w307]
              tunnel: [w306] -> w240 mode=indexing
              n120 = Negate(x=w307) -> (-x=w305:dbl[])
              n121 = Add(x=w304, y=w305) -> (x+y=w306:dbl[])
            }
            n122 = for {
              tunnel: w280 -> [w352] mode=indexing
              tunnel: w270 -> [w355]
              tunnel: [w354] -> w241 mode=indexing
              n123 = Negate(x=w355) -> (-x=w353:dbl[])
              n124 = Add(x=w352, y=w353) -> (x+y=w354:dbl[])
            }
            n125 = case shown="True" w248 {
              tunnel: w278 -> [w318 w332]
              tunnel: [w318 w350] -> w303
              tunnel: [w317 ctlTrialState."no events" ("Trigger events")] -> w254
              tunnel: w238 -> [_ w333]
              tunnel: w239 -> [_ w331]
              tunnel: w240 -> [_ w330]
              tunnel: w241 -> [_ w329]
              tunnel: w250 -> [w317 w328]
              tunnel: w249 -> [_ w320]
              tunnel: w268 -> [_ w324]
              tunnel: w252 -> [_ w325]
              tunnel: [w316 w319] -> w251
              tunnel: w247 -> [_ w323]
              tunnel: w246 -> [_ w322]
              tunnel: w245 -> [_ w321]
              tunnel: w243 -> [w316 w319]
              frame False {
              }
              frame True {
                w343 = "ATI Data" ("group name")
                w344 = enum16{"decimated", "interleaved"}."interleaved" ("data layout (0:decimated)")
                w347 = "Events" ("group name")
                n126 = TDMS Write(0:w325, 1:w344, 5:w343, 7:w324, 9:w333, 11:w332) -> (4:w337:refnum<k34>, 15:w340:errorcluster)  [unwired: 2 out]
                n127 = TDMS Write(0:w337, 1:w344, 5:w343, 7:w323, 9:w331, 11:w340) -> (4:w338:refnum<k34>, 15:w341:errorcluster)  [unwired: 2 out]
                n128 = TDMS Write(0:w338, 1:w344, 5:w343, 7:w322, 9:w330, 11:w341) -> (4:w339:refnum<k34>, 15:w342:errorcluster)  [unwired: 2 out]
                n129 = Build Array(w328) -> (w327:T3[])
                n130 = TDMS Write(0:w339, 1:w344, 5:w343, 7:w321, 9:w329, 11:w342) -> (4:w336:refnum<k34>, 15:w335:errorcluster)  [unwired: 2 out]
                n131 = Add(x=w319, y=w320) -> (x+y=w346:i64)
                n132 = Build Array(w346) -> (w345:i64[])
                n133 = TDMS Write(0:w336, 5:w347, 7:"TriggerATI" ("channel name"), 9:w327, 11:w335) -> (4:w348:refnum<k34>, 15:w349:errorcluster)  [unwired: 1 in, 2 out]
                n134 = TDMS Write(0:w348, 5:w347, 7:"TimeATI" ("channel name"), 9:w345, 11:w349) -> (15:w350:errorcluster)  [unwired: 1 in, 3 out]
              }
            }
            n135 = Bundle(w238) -> (w259:cluster{dbl[][]})  [unwired: 1 in]
            n136 = Bundle(w239) -> (w258:cluster{dbl[][]})  [unwired: 1 in]
            n137 = Bundle(w240) -> (w257:cluster{dbl[][]})  [unwired: 1 in]
            n138 = Bundle(w241) -> (w256:cluster{dbl[][]})  [unwired: 1 in]
            n139 = Build Array(w259, w258, w257, w256) -> (w255:cluster{dbl[][]}[])
          }
          frame False {
            n140 = Index Array(array=w365) -> (element=w363:cluster{"Real Matrix":T4})  [unwired: 1 in]
            n141 = Index Array(array=w383) -> (element=w382:refnum<k21>)  [unwired: 1 in]
            n142 = call-poly <vilib>:"DAQmx Read.vi"("task/channels in"=w382, "error in"=w364) -> ("data"=w387:dbl[][], "error out"=w384:errorcluster)  [unwired: 11 in, 1 out]
            n143 = Unbundle(w363) -> ("Real Matrix"=w380:T4)
            n144 = call-poly <vilib>:"Array To Matrix.vi"("Real 2D Array"=w387) -> ("Real Matrix"=w388:T4)
            n145 = call-poly <vilib>:"A x B.vi"("B"=w388, "A"=w380) -> ("A x B"=w389:T4)  [unwired: 1 out]
            n146 = Index Array(array=w376) -> (element=w362:dbl[])  [unwired: 2 in]
            n147 = call-poly <vilib>:"Matrix To Array.vi"("Real Matrix"=w389) -> ("Real 2D Array"=w386:dbl[][])
            n148 = Transpose 2D Array(2D array=w386) -> (transposed array=w385:dbl[][])
            n149 = for {
              tunnel: w385 -> [w417] mode=indexing
              tunnel: w362 -> [w420]
              tunnel: [w419] -> w357 mode=indexing
              n150 = Negate(x=w420) -> (-x=w418:dbl[])
              n151 = Add(x=w417, y=w418) -> (x+y=w419:dbl[])
            }
            n152 = Tick Count (ms)() -> (millisecond timer value=w367:u32)
            n153 = To Quad Integer(1:w367) -> (0:w366:i64)
            n154 = case shown="True" w371 {
              tunnel: w384 -> [w393 w399]
              tunnel: [w393 w415] -> w390
              tunnel: [w392 ctlTrialState."no events" ("Trigger events")] -> w377
              tunnel: w357 -> [_ w396]
              tunnel: w373 -> [w392 w404]
              tunnel: w372 -> [_ w401]
              tunnel: w381 -> [_ w394]
              tunnel: w375 -> [_ w397]
              tunnel: [w391 w400] -> w374
              tunnel: w370 -> [_ w395]
              tunnel: w369 -> [_ _]
              tunnel: w368 -> [_ _]
              tunnel: w366 -> [w391 w400]
              frame False {
              }
              frame True {
                w412 = "Events" ("group name")
                n155 = Build Array (concatenate)(w394, w395) -> (w398:string[])
                n156 = Build Array(w404) -> (w403:T3[])
                n157 = TDMS Write(0:w397, 1:enum16{"decimated", "interleaved"}."interleaved" ("data layout (0:decimated)"), 5:"ATI Data" ("group name"), 7:w398, 9:w396, 11:w399) -> (4:w407:refnum<k34>, 15:w406:errorcluster)  [unwired: 2 out]
                n158 = Add(x=w400, y=w401) -> (x+y=w411:i64)
                n159 = Build Array(w411) -> (w410:i64[])
                n160 = TDMS Write(0:w407, 5:w412, 7:"TriggerATI" ("channel name"), 9:w403, 11:w406) -> (4:w413:refnum<k34>, 15:w414:errorcluster)  [unwired: 1 in, 2 out]
                n161 = TDMS Write(0:w413, 5:w412, 7:"TimeATI" ("channel name"), 9:w410, 11:w414) -> (15:w415:errorcluster)  [unwired: 1 in, 3 out]
              }
            }
            n162 = Delete From Array(array=w357, length=6, index (col)=0 ("disabled index (col)")) -> (deleted portion=w359:dbl[][], array with subset deleted=w360:dbl[][])  [unwired: 1 in]
            n163 = Bundle(w359) -> (w361:cluster{dbl[][]})  [unwired: 1 in]
            n164 = Bundle(w360) -> (w379:cluster{dbl[][]})  [unwired: 1 in]
            n165 = Build Array(w379, w361) -> (w378:cluster{dbl[][]}[])
          }
        }
        n166 = Add(x=w211, y=w215) -> (x+y=w217:i64)
        n167 = Negate(x=w215) -> (-x=w207:i64)
        n168 = To Double Precision Float(number=w217) -> (double precision float=w214:dbl)
        n169 = Bundle By Name(cluster=w226, "tick pre"=w207, "Trigger events"=w223, "Data"=w195) -> (w228:T2)
        n170 = Index Array(array=w195) -> (element #1=w203:cluster{dbl[][]}, element #2=w202:cluster{dbl[][]}, element #3=w201:cluster{dbl[][]}, element #4=w200:cluster{dbl[][]})  [unwired: 4 in]
        n171 = Reciprocal(x=w214) -> (1/x=w218:dbl)
        n172 = call "Elapsed Time"("Time Target (s)"="Read Cycle Time (s)", "error in (no error)"=w230) -> ("Time has Elapsed"=w231:bool, "error out"=w229:errorcluster)  [unwired: 10 in, 6 out]
        n173 = Multiply(x=1000.0, y=w218) -> (x*y=→"Hz":dbl)
        n174 = case shown="True" w231 {
          tunnel: [_ cluster{"FN":T5, "Data":variant}[] [{"FN"=enum."SEND2MAIN", "Data"=variant}] ("QFNs")] -> w232
          frame False {
          }
          frame True {
          }
        }
        n175 = Unbundle(w203) -> (→"ATI plot 1":dbl[][])
        n176 = Unbundle(w202) -> (→"ATI plot 2":dbl[][])
        n177 = Unbundle(w201) -> (→"ATI plot 3":dbl[][])
        n178 = Unbundle(w200) -> (→"ATI plot 4":dbl[][])
        n179 = Build Array (concatenate)(w232, cluster{"FN":T5, "Data":variant}[] [{"FN"=enum."IDLE", "Data"=variant}] ("QFNs")) -> (w233:cluster{"FN":T5, "Data":variant}[])
      }
      frame "CALIB Load" {
        n180 = Unbundle By Name(w423) -> ("UShape?"=w422:bool)
        n181 = case shown="False" w422 {
          tunnel: [w432 w446] -> w424
          frame True {
            n182 = Unbundle By Name("Calib files - UShape") -> ("Calibration Files 1"=w430:path[], "Calibration Files 2"=w429:path[], "Calibration Files 3"=w428:path[], "Calibration Files 4"=w427:path[])
            n183 = call "CalibMatrix (SubVI).vi"("Calibration Files"=w430) -> ("Calib Matrix"=w444:dbl[][])  [unwired: 1 out]
            n184 = call "CalibMatrix (SubVI).vi"("Calibration Files"=w429) -> ("Calib Matrix"=w443:dbl[][])  [unwired: 1 out]
            n185 = call "CalibMatrix (SubVI).vi"("Calibration Files"=w428) -> ("Calib Matrix"=w442:dbl[][])  [unwired: 1 out]
            n186 = call "CalibMatrix (SubVI).vi"("Calibration Files"=w427) -> ("Calib Matrix"=w441:dbl[][])  [unwired: 1 out]
            n187 = call-poly <vilib>:"Array To Matrix.vi"("Real 2D Array"=w444) -> ("Real Matrix"=w440:T4)
            n188 = call-poly <vilib>:"Array To Matrix.vi"("Real 2D Array"=w443) -> ("Real Matrix"=w438:T4)
            n189 = call-poly <vilib>:"Array To Matrix.vi"("Real 2D Array"=w442) -> ("Real Matrix"=w437:T4)
            n190 = call-poly <vilib>:"Array To Matrix.vi"("Real 2D Array"=w441) -> ("Real Matrix"=w436:T4)
            n191 = Bundle("Real Matrix"=w440) -> (w439:cluster{"Real Matrix":T4})  [unwired: 1 in]
            n192 = Bundle("Real Matrix"=w438) -> (w435:cluster{"Real Matrix":T4})  [unwired: 1 in]
            n193 = Bundle("Real Matrix"=w437) -> (w434:cluster{"Real Matrix":T4})  [unwired: 1 in]
            n194 = Bundle("Real Matrix"=w436) -> (w433:cluster{"Real Matrix":T4})  [unwired: 1 in]
            n195 = Build Array(w439, w435, w434, w433) -> (w432:cluster{"Real Matrix":T4}[])
          }
          frame False {
            n196 = call "CalibMatrix (SubVI).vi"("Calibration Files"="Calib Files - TShape") -> ("Calib Matrix"=w449:dbl[][])  [unwired: 1 out]
            n197 = call-poly <vilib>:"Array To Matrix.vi"("Real 2D Array"=w449) -> ("Real Matrix"=w448:T4)
            n198 = Bundle("Real Matrix"=w448) -> (w447:cluster{"Real Matrix":T4})  [unwired: 1 in]
            n199 = Build Array(w447) -> (w446:cluster{"Real Matrix":T4}[])
          }
        }
        n200 = Bundle By Name(cluster=w423, "CalibMatrix"=w424) -> (w426:T2)
      }
      frame "BIAS" {
        n201 = Unbundle By Name(w451) -> ("UShape?"=w450:bool)
        n202 = case shown="False" w450 {
          tunnel: w451 -> [w495 w517]
          tunnel: [w471 w511] -> w454
          tunnel: w453 -> [w466 w505]
          tunnel: [w465 w507] -> w452
          frame True {
            n203 = Unbundle By Name(w495) -> ("CalibMatrix"=w464:cluster{"Real Matrix":T4}[], "DAQmx"=w496:refnum<k21>[])
            n204 = Index Array(array=w496) -> (element #1=w470:refnum<k21>, element #2=w469:refnum<k21>, element #3=w468:refnum<k21>, element #4=w467:refnum<k21>)  [unwired: 4 in]
            n205 = Index Array(array=w464) -> (element #1=w463:cluster{"Real Matrix":T4}, element #2=w461:cluster{"Real Matrix":T4}, element #3=w460:cluster{"Real Matrix":T4}, element #4=w459:cluster{"Real Matrix":T4})  [unwired: 4 in]
            n206 = call-poly <vilib>:"DAQmx Read.vi"("task/channels in"=w470, "error in"=w466) -> ("data"=w481:dbl[][], "error out"=w476:errorcluster)  [unwired: 11 in, 1 out]
            n207 = Unbundle(w463) -> ("Real Matrix"=w462:T4)
            n208 = Unbundle(w461) -> ("Real Matrix"=w458:T4)
            n209 = Unbundle(w460) -> ("Real Matrix"=w457:T4)
            n210 = Unbundle(w459) -> ("Real Matrix"=w456:T4)
            n211 = call-poly <vilib>:"DAQmx Read.vi"("task/channels in"=w469, "error in"=w476) -> ("data"=w488:dbl[][], "error out"=w477:errorcluster)  [unwired: 11 in, 1 out]
            n212 = call-poly <vilib>:"DAQmx Read.vi"("task/channels in"=w468, "error in"=w477) -> ("data"=w489:dbl[][], "error out"=w478:errorcluster)  [unwired: 11 in, 1 out]
            n213 = call-poly <vilib>:"DAQmx Read.vi"("task/channels in"=w467, "error in"=w478) -> ("data"=w490:dbl[][], "error out"=w465:errorcluster)  [unwired: 11 in, 1 out]
            n214 = call-poly <vilib>:"Array To Matrix.vi"("Real 2D Array"=w481) -> ("Real Matrix"=w479:T4)
            n215 = call-poly <vilib>:"Array To Matrix.vi"("Real 2D Array"=w488) -> ("Real Matrix"=w483:T4)
            n216 = call-poly <vilib>:"Array To Matrix.vi"("Real 2D Array"=w489) -> ("Real Matrix"=w484:T4)
            n217 = call-poly <vilib>:"Array To Matrix.vi"("Real 2D Array"=w490) -> ("Real Matrix"=w487:T4)
            n218 = call-poly <vilib>:"A x B.vi"("B"=w479, "A"=w462) -> ("A x B"=w480:T4)  [unwired: 1 out]
            n219 = call-poly <vilib>:"A x B.vi"("B"=w483, "A"=w458) -> ("A x B"=w482:T4)  [unwired: 1 out]
            n220 = call-poly <vilib>:"A x B.vi"("B"=w484, "A"=w457) -> ("A x B"=w485:T4)  [unwired: 1 out]
            n221 = call-poly <vilib>:"A x B.vi"("B"=w487, "A"=w456) -> ("A x B"=w486:T4)  [unwired: 1 out]
            n222 = call-poly <vilib>:"Matrix To Array.vi"("Real Matrix"=w480) -> ("Real 2D Array"=w491:dbl[][])
            n223 = call-poly <vilib>:"Matrix To Array.vi"("Real Matrix"=w482) -> ("Real 2D Array"=w492:dbl[][])
            n224 = call-poly <vilib>:"Matrix To Array.vi"("Real Matrix"=w485) -> ("Real 2D Array"=w493:dbl[][])
            n225 = call-poly <vilib>:"Matrix To Array.vi"("Real Matrix"=w486) -> ("Real 2D Array"=w494:dbl[][])
            n226 = for {
              tunnel: w491 -> [w504] mode=indexing
              tunnel: [w503] -> w475 mode=indexing
              n227 = call-poly <vilib>:"Mean.vi"("X"=w504) -> ("mean"=w503:dbl)  [unwired: 1 out]
            }
            n228 = for {
              tunnel: w492 -> [w502] mode=indexing
              tunnel: [w501] -> w474 mode=indexing
              n229 = call-poly <vilib>:"Mean.vi"("X"=w502) -> ("mean"=w501:dbl)  [unwired: 1 out]
            }
            n230 = for {
              tunnel: w493 -> [w500] mode=indexing
              tunnel: [w499] -> w473 mode=indexing
              n231 = call-poly <vilib>:"Mean.vi"("X"=w500) -> ("mean"=w499:dbl)  [unwired: 1 out]
            }
            n232 = for {
              tunnel: w494 -> [w498] mode=indexing
              tunnel: [w497] -> w472 mode=indexing
              n233 = call-poly <vilib>:"Mean.vi"("X"=w498) -> ("mean"=w497:dbl)  [unwired: 1 out]
            }
            n234 = Build Array(w475, w474, w473, w472) -> (w471:dbl[][])
          }
          frame False {
            n235 = Unbundle By Name(w517) -> ("CalibMatrix"=w510:cluster{"Real Matrix":T4}[], "DAQmx"=w518:refnum<k21>[])
            n236 = Index Array(array=w510) -> (element=w509:cluster{"Real Matrix":T4})  [unwired: 1 in]
            n237 = Index Array(array=w518) -> (element=w506:refnum<k21>)  [unwired: 1 in]
            n238 = call-poly <vilib>:"DAQmx Read.vi"("task/channels in"=w506, "error in"=w505) -> ("data"=w515:dbl[][], "error out"=w507:errorcluster)  [unwired: 11 in, 1 out]
            n239 = Unbundle(w509) -> ("Real Matrix"=w508:T4)
            n240 = call-poly <vilib>:"Array To Matrix.vi"("Real 2D Array"=w515) -> ("Real Matrix"=w513:T4)
            n241 = call-poly <vilib>:"A x B.vi"("B"=w513, "A"=w508) -> ("A x B"=w514:T4)  [unwired: 1 out]
            n242 = call-poly <vilib>:"Matrix To Array.vi"("Real Matrix"=w514) -> ("Real 2D Array"=w516:dbl[][])
            n243 = for {
              tunnel: w516 -> [w520] mode=indexing
              tunnel: [w519] -> w512 mode=indexing
              n244 = call-poly <vilib>:"Mean.vi"("X"=w520) -> ("mean"=w519:dbl)  [unwired: 1 out]
            }
            n245 = Build Array(w512) -> (w511:dbl[][])
          }
        }
        n246 = Bundle By Name(cluster=w451, "Bias"=w454) -> (w455:T2)
      }
      frame "SEND2MAIN" {
        n247 = Unbundle By Name(w526) -> ("MAIN"=w525:refnum<queue>, "Data"=w524:cluster{dbl[][]}[])
        n248 = To Variant(anything=w524) -> (Variant=w523:variant)
        n249 = Bundle By Name(cluster=cluster{"STATE":T6, "Data":variant} {"STATE"=enum."Get ATI", "Data"=variant} ("element"), "Data"=w523) -> (w521:cluster{"STATE":T6, "Data":variant})
        n250 = Enqueue Element(queue=w525, element=w521, error in (no error)=w528) -> (error out=w527:errorcluster)  [unwired: 1 in, 2 out]
      }
      frame "READY" {
        n251 = Variant To Data(error in=w533, type=T9 {"recording?"=FALSE, "tdms file"=refnum} ("output cluster"), Variant=w540) -> (data=w537:T9, error out=w539:errorcluster)
        n252 = Unbundle By Name(w537) -> ("recording?"=w529:bool, "tdms file"=w530:refnum<k34>)
        n253 = Refnum to Path(1:w530) -> (0:→"save file":path)
        n254 = Tick Count (ms)() -> (millisecond timer value=w542:u32)
        n255 = To Quad Integer(1:w542) -> (0:w541:i64)
        n256 = Negate(x=w541) -> (-x=w536:i64)
        n257 = Bundle By Name(cluster=w535, "tick ini"=w536, "recording?"=w529, "Trigger events"=ctlTrialState."ready", "ATI"=w530) -> (w544:T2)
      }
      frame "TRIGGER" {
        n258 = Variant To Data(error in=w551, type=ctlTrialState."no events" ("Trigger events"), Variant=w549) -> (data=w545:T3, error out=w550:errorcluster)
        n259 = Bundle By Name(cluster=w547, "Trigger events"=w545) -> (w548:T2)
      }
      frame "END" {
        n260 = Unbundle By Name(w555) -> ("MAIN"=w556:refnum<queue>)
        n261 = Enqueue Element(queue=w556, element=cluster{"STATE":T6, "Data":variant} {"STATE"=enum."End ATI", "Data"=variant}, error in (no error)=w553) -> (error out=w552:errorcluster)  [unwired: 1 in, 2 out]
        n262 = Bundle By Name(cluster=w555, "recording?"=FALSE, "Trigger events"=ctlTrialState."no events") -> (w559:T2)
      }
      frame "ERROR" {
        n263 = call <vilib>:"General Error Handler.vi"("error in (no error)"=w560) -> ()  [unwired: 10 in, 5 out]
        n264 = call "Error Clear.vi"("wait(ms)"=u32 5000, "error in"=w560) -> ("error in (no error)"=w562:errorcluster)  [unwired: 6 in]
      }
      frame "EXIT" {
        n265 = Unbundle By Name(w566) -> ("UShape?"=w564:bool, "DAQmx"=w565:refnum<k21>[])
        n266 = case shown="False" w564 {
          tunnel: [w576 w583] -> w568
          tunnel: w567 -> [w575 w580]
          tunnel: w565 -> [w574 w582]
          frame True {
            n267 = Index Array(array=w574) -> (element #1=w570:refnum<k21>, element #2=w571:refnum<k21>, element #3=w573:refnum<k21>, element #4=w572:refnum<k21>)  [unwired: 4 in]
            n268 = call <vilib>:"DAQmx Clear Task.vi"("task in"=w572, "error in"=w575) -> ("error out"=w579:errorcluster)  [unwired: 13 in]
            n269 = call <vilib>:"DAQmx Clear Task.vi"("task in"=w573, "error in"=w579) -> ("error out"=w578:errorcluster)  [unwired: 13 in]
            n270 = call <vilib>:"DAQmx Clear Task.vi"("task in"=w571, "error in"=w578) -> ("error out"=w577:errorcluster)  [unwired: 13 in]
            n271 = call <vilib>:"DAQmx Clear Task.vi"("task in"=w570, "error in"=w577) -> ("error out"=w576:errorcluster)  [unwired: 13 in]
          }
          frame False {
            n272 = Index Array(array=w582) -> (element=w581:refnum<k21>)  [unwired: 1 in]
            n273 = call <vilib>:"DAQmx Clear Task.vi"("task in"=w581, "error in"=w580) -> ("error out"=w583:errorcluster)  [unwired: 13 in]
          }
        }
        n274 = case shown="No Error" w568 {
          selector: w568 -> [w584 w586]
          tunnel: [w584 w586] -> w569
          frame No Error {
            n275 = global write "GLOBAL -MAIN.vi" "EXIT"(TRUE ("EXIT")) -> ()
          }
          frame Error {
          }
        }
      }
    }
    n276 = call "QSM Queue Mgr SubVI ATI.vi"("QRef"=w24, "Error IN"=w27, "FNs"=w25, "QSTATES"=w23) -> ("Error OUT"=w26:errorcluster)  [unwired: 4 in]
  }
  n277 = Release Queue(queue=w5, force destroy? (F)=TRUE, error in (no error)=w1) -> ()  [unwired: 3 out]
